vi "control v3.vi"(0 "Contraste":dbl, 1 "Ajuste ON?":bool=TRUE, 2 "Control ON?":bool=TRUE, 5 "Arreglo de Salida":dbl[](array[numeric]), 7 "Señal de Control IN":dbl[](array[numeric]), 9 "Parametros Actuales":T2, 11 "Parametros Iniciales":T2, 12 "Parametros Control":T3) -> (4 "Control Case OUT":T1 items=["00 - Promedio Inicial", "01 - Genera señal aleatoria", "02 - Incrementa t0", "03 - Promedia buen t0", "04 - Inicializa Amplitud", "05 - Incrementa Amplitud", "06 - Promedia buena Amplitud", "07 - Inicializa Sigma", "08 - Incrementa Sigma", "09 - Promedia buen Sigma", "10 - Actualiza mejor señal", "11 - Control ON, Ajuste OFF", "12 - Control OFF"], 6 "Contraste Promedio":dbl, 8 "Señal de Control OUT":dbl[](array[numeric]), 10 "Mejores Parametros OUT":T2)   [LabVIEW 2010]
uses:
  CaseControl.ctl
  <vilib>/Analysis/NI_AALBase.lvlib
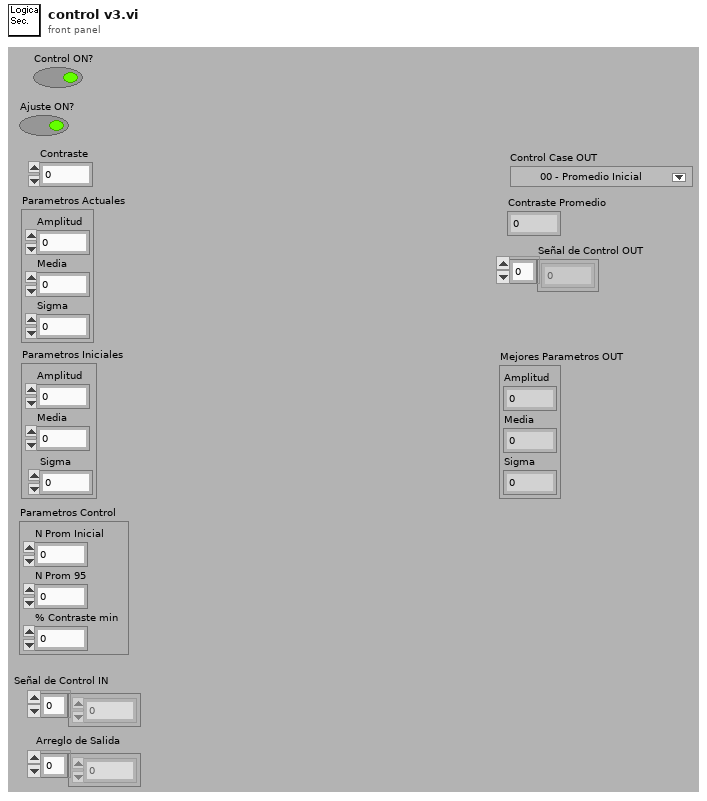
[diagram p1: front panel]
types:
  T1 = typedef "CaseControl.ctl" = u32
  T2 = cluster{"Amplitud":dbl, "Media":dbl, "Sigma":dbl}
  T3 = cluster{"N Prom Inicial":u32, "N Prom 95":u32, "% Contraste min":dbl}
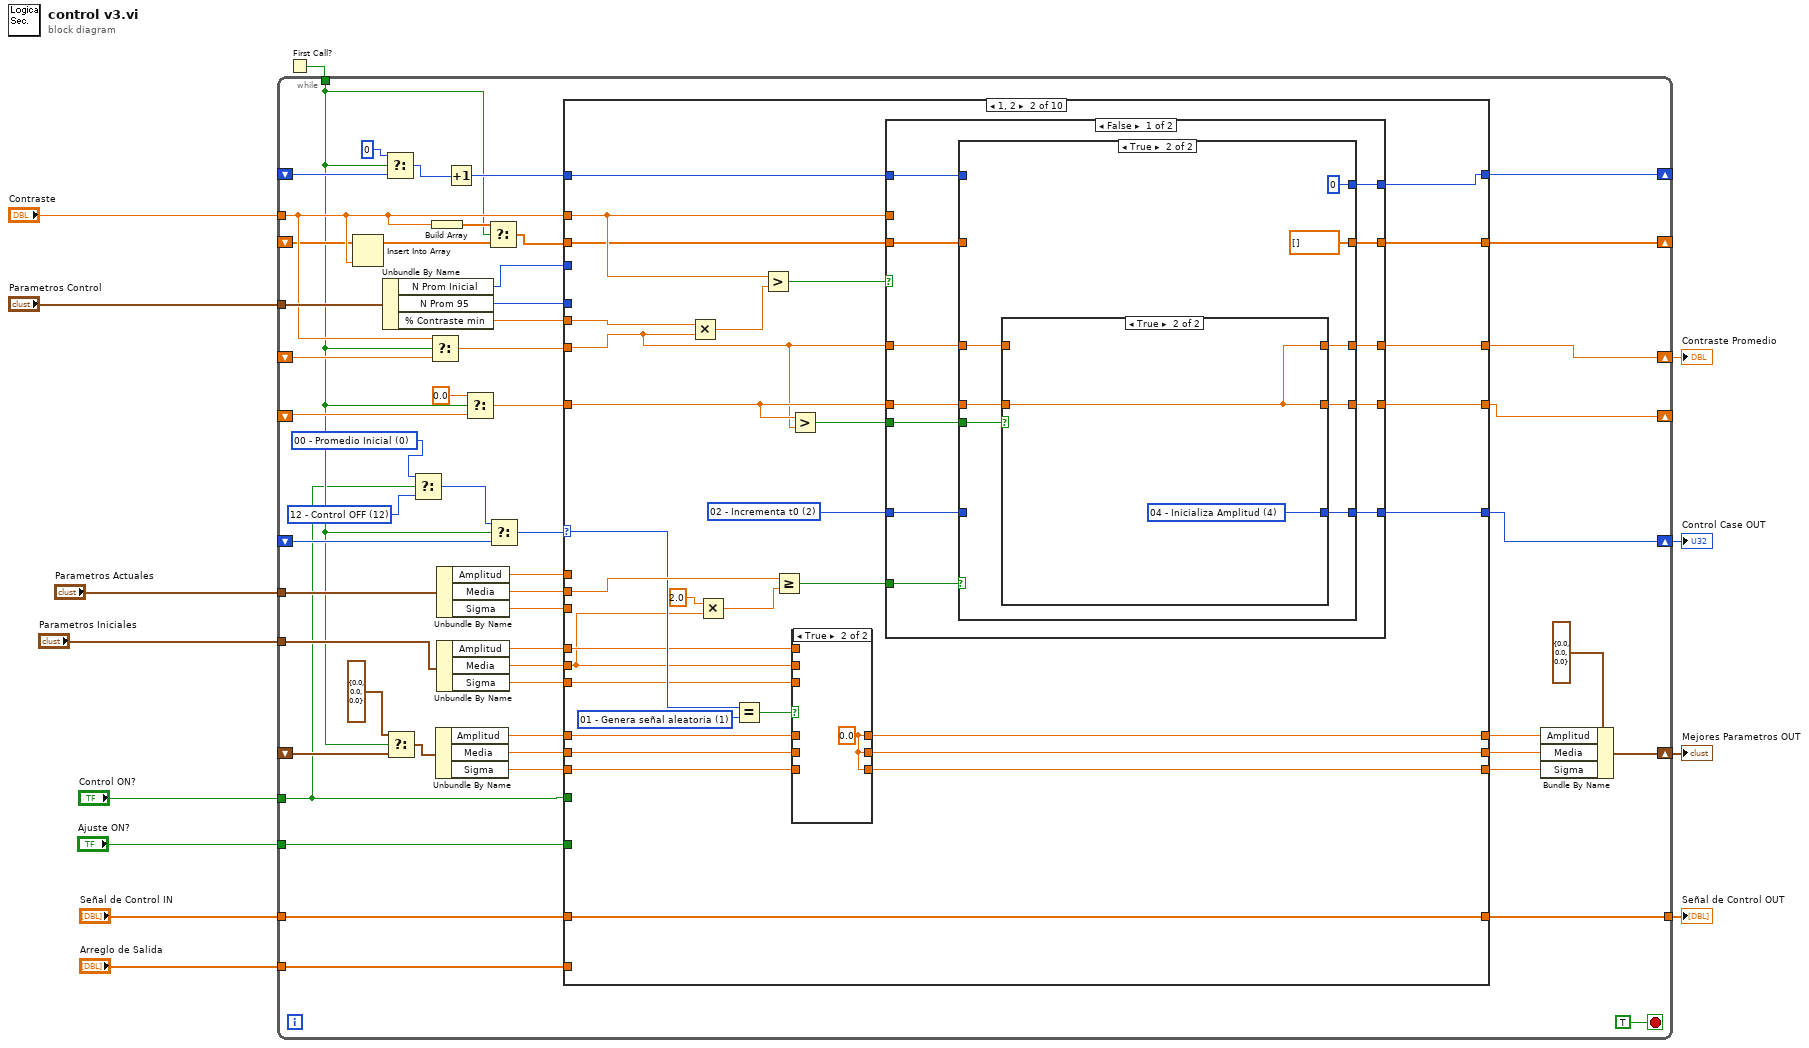
[diagram p0: block diagram]
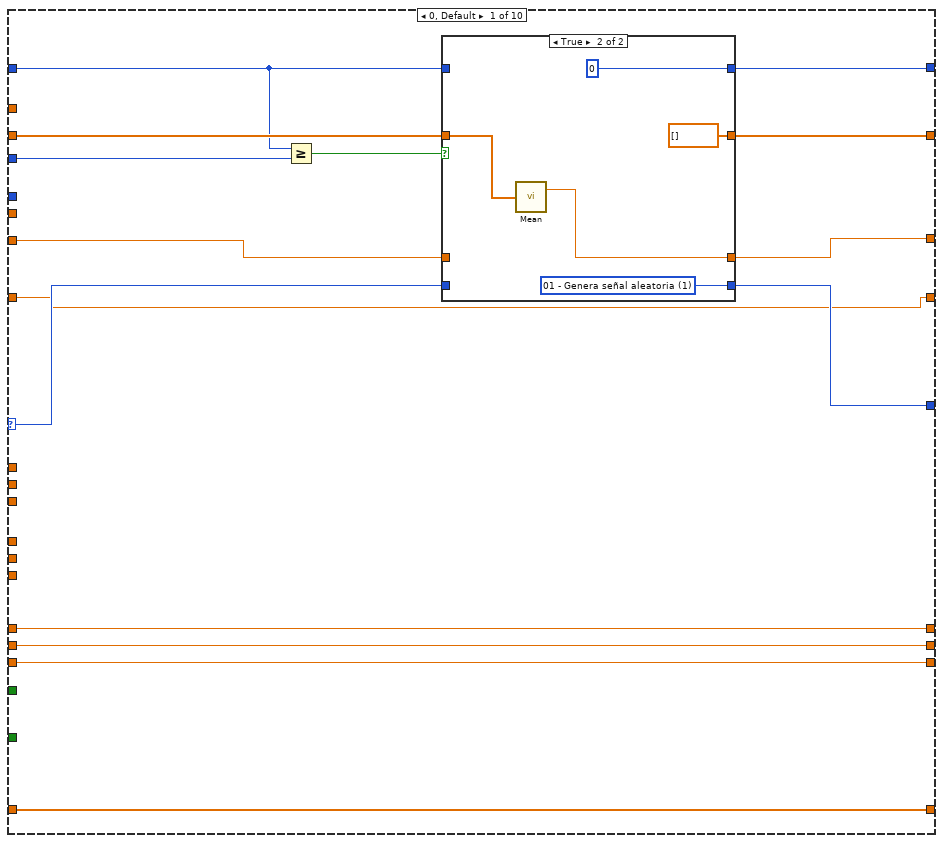
[diagram p2: hidden frame]
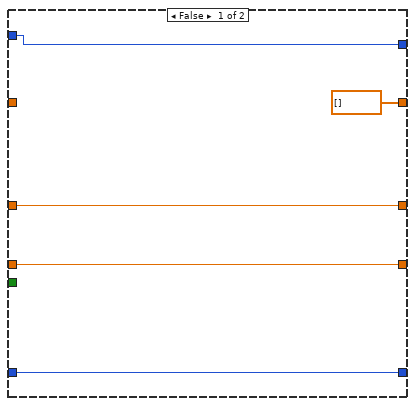
[diagram p5: hidden frame]
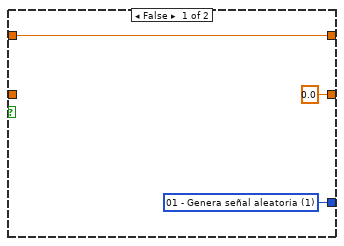
[diagram p6: hidden frame]
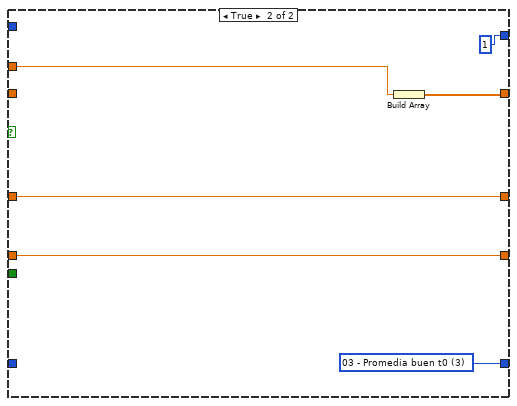
[diagram p7: hidden frame]
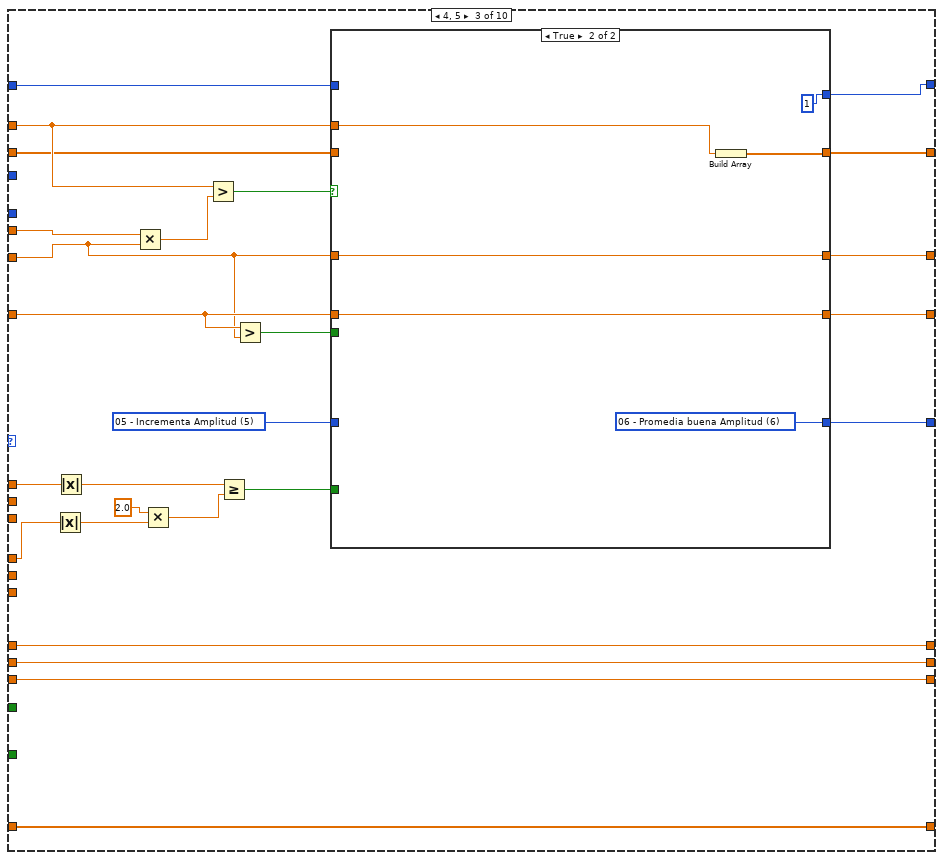
[diagram p8: hidden frame]
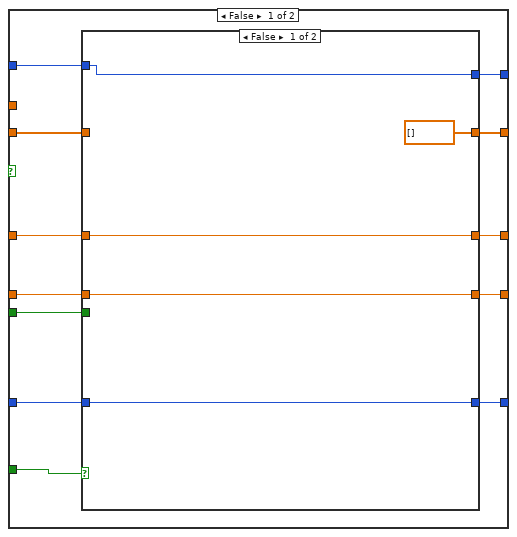
[diagram p9: hidden frame]
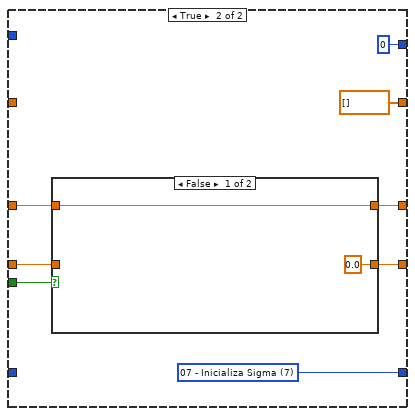
[diagram p10: hidden frame]
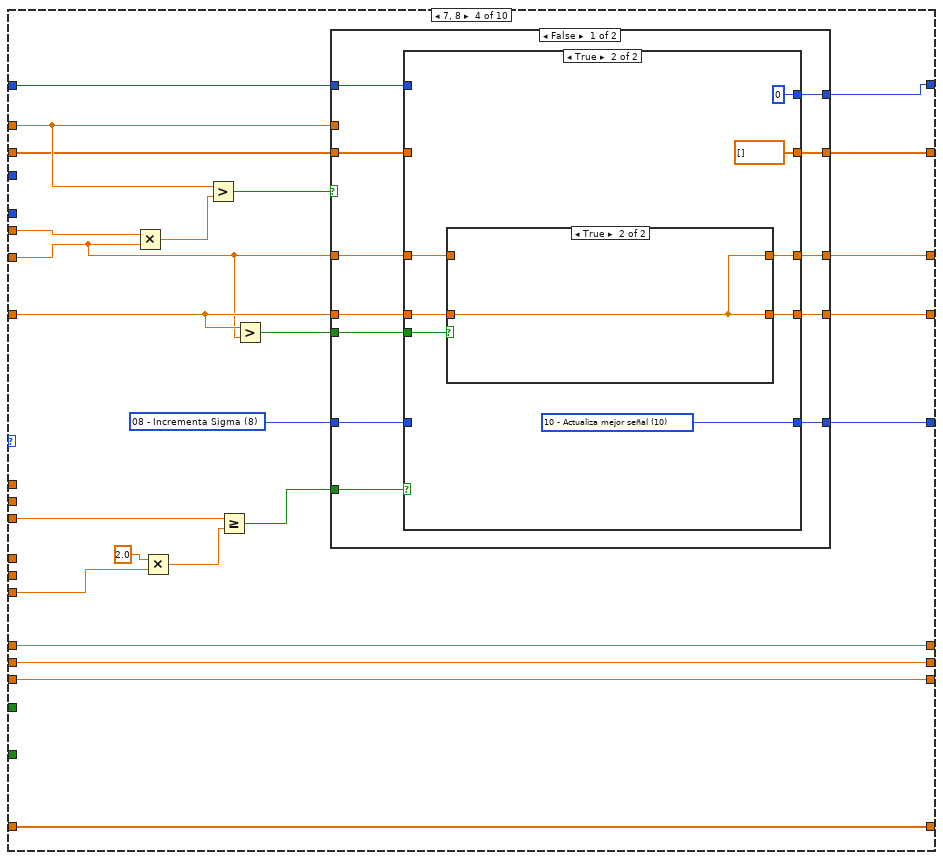
[diagram p12: hidden frame]
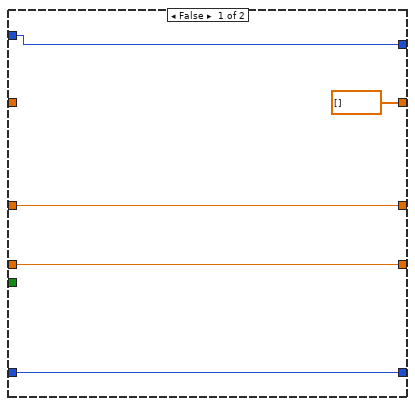
[diagram p13: hidden frame]
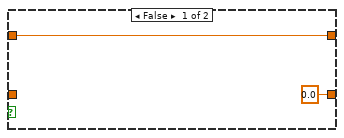
[diagram p14: hidden frame]
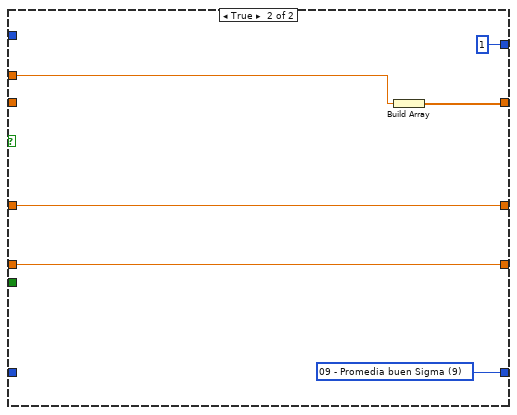
[diagram p15: hidden frame]
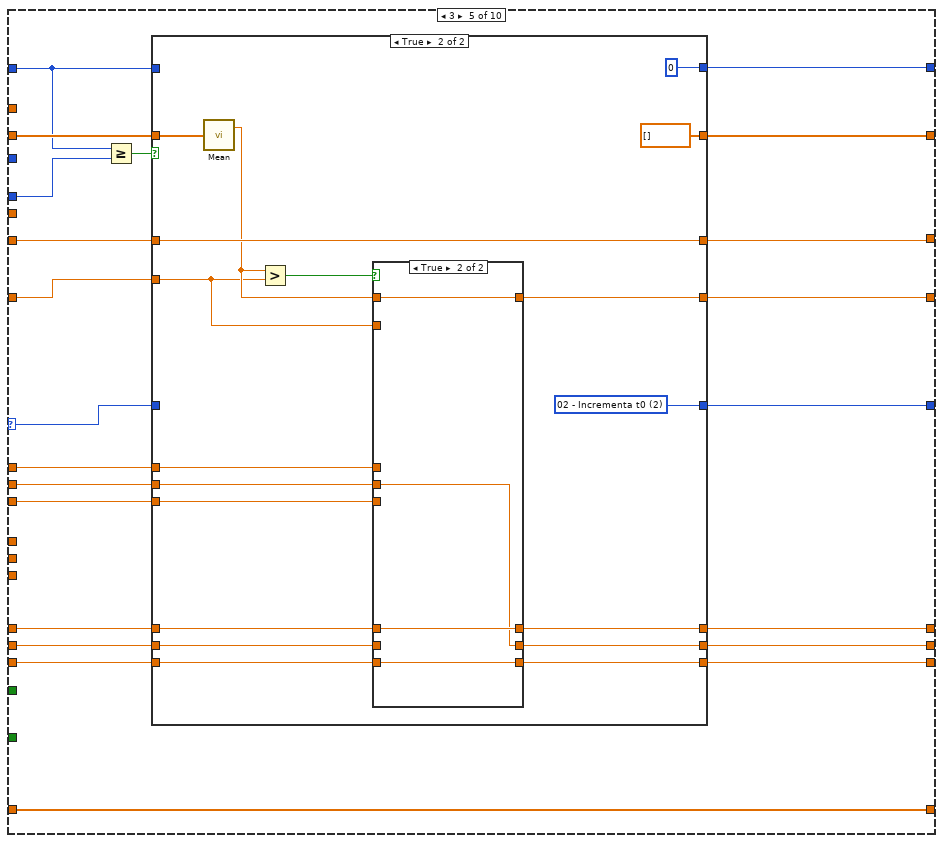
[diagram p16: hidden frame]
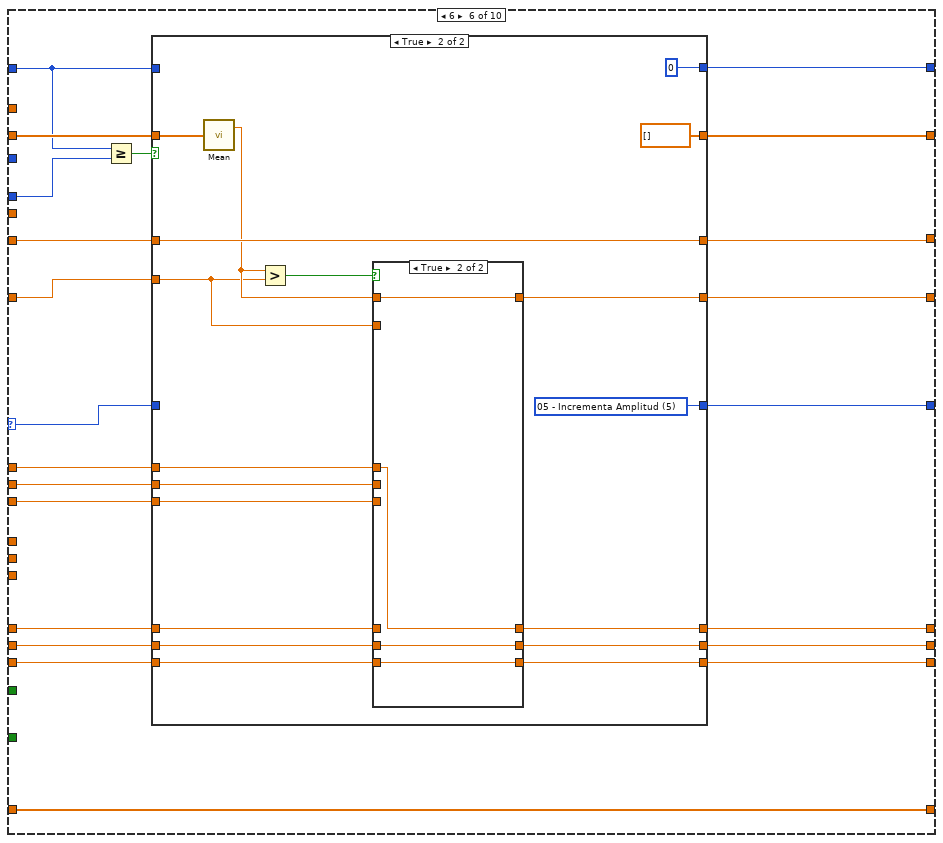
[diagram p19: hidden frame]
diagram:
  n1 = First Call?() -> (First Call?: T/F=w13:bool)
  n2 = while {
    tunnel: w13 -> [w22]
    tunnel: "Contraste" -> [w51]
    tunnel: "Parametros Control" -> [w66]
    shift-right: [w52] -> w3
    shift-left: _ -> [w54]
    shift-right: [w63] -> _
    shift-left: _ -> [w65]
    shift-right: [w60] -> _
    shift-left: _ -> [w48]
    shift-right: [w59] -> w2
    shift-left: _ -> [w58]
    tunnel: "Parametros Actuales" -> [w39]
    tunnel: "Parametros Iniciales" -> [w38]
    shift-right: [w34] -> w8
    shift-left: _ -> [w23]
    shift-right: [w26] -> _
    shift-left: _ -> [w29]
    tunnel: "Señal de Control IN" -> [w21]
    tunnel: "Arreglo de Salida" -> [w20]
    tunnel: [w19] -> w5
    tunnel: "Ajuste ON?" -> [w18]
    tunnel: "Control ON?" -> [w16]
    stop <- TRUE stop-if-true
    w14 = T1 0 items=["00 - Promedio Inicial", "01 - Genera señal aleatoria", "02 - Incrementa t0", "03 - Promedia buen t0", "04 - Inicializa Amplitud", "05 - Incrementa Amplitud", "06 - Promedia buena Amplitud", "07 - Inicializa Sigma", "08 - Incrementa Sigma", "09 - Promedia buen Sigma", "10 - Actualiza mejor señal", "11 - Control ON, Ajuste OFF", "12 - Control OFF"] ("f")
    w15 = T1 12 items=["00 - Promedio Inicial", "01 - Genera señal aleatoria", "02 - Incrementa t0", "03 - Promedia buen t0", "04 - Inicializa Amplitud", "05 - Incrementa Amplitud", "06 - Promedia buena Amplitud", "07 - Inicializa Sigma", "08 - Incrementa Sigma", "09 - Promedia buen Sigma", "10 - Actualiza mejor señal", "11 - Control ON, Ajuste OFF", "12 - Control OFF"] ("f")
    n3 = Insert Into Array(array=w48, new element=w51) -> (w49:dbl[])  [unwired: 1 in]
    n4 = Unbundle By Name(w66) -> ("N Prom Inicial"=w62:u32, "N Prom 95"=w47:u32, "% Contraste min"=w46:dbl)
    n5 = Select(t=u32 0, s=w22, f=w65) -> (s? t:f=w56:u32)
    n6 = Select(t=T2 {"Amplitud"=0.0, "Media"=0.0, "Sigma"=0.0} ("Parametros Iniciales 2"), s=w22, f=w23) -> (s? t:f=w25:T2)
    n7 = Select(t=w14, s=w16, f=w15) -> (s? t:f=w17:T1)
    n8 = Select(t=w51, s=w22, f=w58) -> (s? t:f=w57:dbl)
    n9 = Build Array(w51) -> (w61:dbl[])
    n10 = Unbundle By Name(w25) -> ("Amplitud"=w37:dbl, "Media"=w36:dbl, "Sigma"=w35:dbl)
    n11 = Unbundle By Name(w39) -> ("Amplitud"=w45:dbl, "Media"=w44:dbl, "Sigma"=w43:dbl)
    n12 = Unbundle By Name(w38) -> ("Amplitud"=w42:dbl, "Media"=w41:dbl, "Sigma"=w40:dbl)
    n13 = Increment(x=w56) -> (x+1=w55:u32)
    n14 = Select(t=0.0, s=w22, f=w29) -> (s? t:f=w27:dbl)
    n15 = Select(t=w61, s=w22, f=w49) -> (s? t:f=w50:dbl[])
    n16 = Select(t=w17, s=w22, f=w54) -> (s? t:f=w53:T1)
    n17 = case shown="1, 2" w53 {
      selector: w53 -> [w75 w103 _ _ w297 w353 w409 _ _ _]
      tunnel: w51 -> [_ w116 w182 w240 _ _ _ _ _ _]
      tunnel: [w77 w107 w174 w232 w300 w356 w412 u32 0 ("t") w467 u32 0 ("t")] -> w63
      tunnel: w62 -> [w82 _ _ _ _ _ _ _ _ _]
      tunnel: [w73 w117 w183 w241 w296 w352 w408 w455 w469 w481] -> w52
      tunnel: w50 -> [w81 w114 w180 w238 w302 w358 w414 w451 w466 w484]
      tunnel: [w74 w115 w181 w239 w301 w357 w413 w451 w466 w484] -> w60
      tunnel: [w78 w118 w184 w242 w293 w349 w405 w450 w465 w483] -> w59
      tunnel: w57 -> [w79 w110 w176 w234 w295 w351 w407 w450 _ _]
      tunnel: w55 -> [w76 w106 w173 w231 w299 w355 w411 _ w467 _]
      tunnel: w47 -> [_ _ _ _ w298 w354 w410 _ _ _]
      tunnel: w46 -> [_ w120 w186 w244 _ _ _ _ _ _]
      tunnel: w45 -> [_ _ w168 _ w292 w348 w404 _ _ _]
      tunnel: w44 -> [_ w108 _ _ w291 w347 w403 _ _ _]
      tunnel: w43 -> [_ _ _ w226 w290 w346 w402 _ _ _]
      tunnel: w42 -> [_ w98 w165 _ _ _ _ _ _ _]
      tunnel: w41 -> [_ w97 _ _ _ _ _ _ _ _]
      tunnel: w40 -> [_ w96 _ w225 _ _ _ _ _ _]
      tunnel: w37 -> [w71 w101 w171 w229 w289 w345 w401 w463 w474 w476]
      tunnel: w36 -> [w70 w100 w170 w228 w288 w344 w400 w462 w473 w477]
      tunnel: w35 -> [w69 w99 w169 w227 w287 w343 w399 w461 w472 w478]
      tunnel: [w71 w95 w171 w229 w285 w341 w397 w463 w474 w476] -> w32
      tunnel: [w70 w94 w170 w228 w283 w339 w395 w462 w473 w477] -> w31
      tunnel: [w69 w93 w169 w227 w284 w340 w396 w461 w472 w478] -> w30
      tunnel: w27 -> [w72 w111 w177 w235 w294 w350 w406 _ _ _]
      tunnel: [w72 w112 w178 w236 w286 w342 w398 0.0 ("mean") 0.0 ("t") 0.0 ("t")] -> w26
      tunnel: w21 -> [w68 w92 w164 w224 w282 w338 w394 w457 w475 w479]
      tunnel: w20 -> [_ _ _ _ _ _ _ w456 _ _]
      tunnel: [w68 w92 w164 w224 w282 w338 w394 w458 w475 w479] -> w19
      tunnel: w18 -> [_ _ _ _ _ _ _ w453 w468 _]
      tunnel: w16 -> [_ _ _ _ _ _ _ _ _ w480]
      frame 0, Default {
        n18 = Greater Or Equal?(x=w76, y=w82) -> (x >= y?=w80:bool)
        n19 = case shown="True" w80 {
          tunnel: w81 -> [w83 w88]
          tunnel: [w86 w91] -> w78
          tunnel: w79 -> [w86 _]
          tunnel: w76 -> [w85 _]
          tunnel: [w85 u32 0 ("t")] -> w77
          tunnel: [w84 w89] -> w73
          tunnel: w75 -> [w84 _]
          tunnel: [w83 dbl[] []] -> w74
          frame False {
          }
          frame True {
            w89 = T1 1 items=["00 - Promedio Inicial", "01 - Genera señal aleatoria", "02 - Incrementa t0", "03 - Promedia buen t0", "04 - Inicializa Amplitud", "05 - Incrementa Amplitud", "06 - Promedia buena Amplitud", "07 - Inicializa Sigma", "08 - Incrementa Sigma", "09 - Promedia buen Sigma", "10 - Actualiza mejor señal", "11 - Control ON, Ajuste OFF", "12 - Control OFF"] ("ControlCase")
            n20 = call <vilib>:"Mean.vi"("X"=w88) -> ("mean"=w91:dbl)  [unwired: 1 out]
          }
        }
      }
      frame 1, 2 {
        w102 = T1 1 items=["00 - Promedio Inicial", "01 - Genera señal aleatoria", "02 - Incrementa t0", "03 - Promedia buen t0", "04 - Inicializa Amplitud", "05 - Incrementa Amplitud", "06 - Promedia buena Amplitud", "07 - Inicializa Sigma", "08 - Incrementa Sigma", "09 - Promedia buen Sigma", "10 - Actualiza mejor señal", "11 - Control ON, Ajuste OFF", "12 - Control OFF"] ("y")
        w105 = T1 2 items=["00 - Promedio Inicial", "01 - Genera señal aleatoria", "02 - Incrementa t0", "03 - Promedia buen t0", "04 - Inicializa Amplitud", "05 - Incrementa Amplitud", "06 - Promedia buena Amplitud", "07 - Inicializa Sigma", "08 - Incrementa Sigma", "09 - Promedia buen Sigma", "10 - Actualiza mejor señal", "11 - Control ON, Ajuste OFF", "12 - Control OFF"] ("ControlCase")
        n21 = Multiply(x=w120, y=w110) -> (x*y=w119:dbl)
        n22 = Multiply(x=2.0, y=w97) -> (x*y=w122:dbl)
        n23 = Equal?(x=w103, y=w102) -> (x = y?=w104:bool)
        n24 = Greater?(x=w116, y=w119) -> (0:w121:bool)
        n25 = Greater Or Equal?(x=w108, y=w122) -> (x >= y?=w113:bool)
        n26 = Greater?(x=w111, y=w110) -> (0:w109:bool)
        n27 = case shown="True" w104 {
          tunnel: [w126 w127] -> w95
          tunnel: w101 -> [w126 _]
          tunnel: [w125 w127] -> w94
          tunnel: w100 -> [w125 _]
          tunnel: [w124 w127] -> w93
          tunnel: w99 -> [w124 _]
          tunnel: w98 -> [_ _]
          tunnel: w97 -> [_ _]
          tunnel: w96 -> [_ _]
          frame False {
          }
          frame True {
            w127 = 0.0 ("Amplitud")
          }
        }
        n28 = case shown="False" w121 {
          tunnel: [w134 w160] -> w118
          tunnel: w110 -> [w133 w160]
          tunnel: [w138 w163] -> w117
          tunnel: w105 -> [w137 _]
          tunnel: w116 -> [_ w161]
          tunnel: [w136 w162] -> w115
          tunnel: w114 -> [w135 _]
          tunnel: w113 -> [w139 _]
          tunnel: w111 -> [w132 w159]
          tunnel: [w131 w159] -> w112
          tunnel: w109 -> [w130 _]
          tunnel: [w129 u32 1] -> w107
          tunnel: w106 -> [w128 _]
          frame False {
            n29 = case shown="True" w139 {
              tunnel: [w144 w151] -> w138
              tunnel: w137 -> [w144 _]
              tunnel: [dbl[] [] dbl[] []] -> w136
              tunnel: w135 -> [_ _]
              tunnel: [w142 w150] -> w134
              tunnel: w133 -> [w142 w147]
              tunnel: w132 -> [w141 w149]
              tunnel: [w141 w148] -> w131
              tunnel: w130 -> [_ w152]
              tunnel: [w140 u32 0] -> w129
              tunnel: w128 -> [w140 _]
              frame False {
              }
              frame True {
                n30 = case shown="True" w152 {
                  tunnel: [w155 w157] -> w151
                  tunnel: [w154 w156] -> w150
                  tunnel: w149 -> [_ w156]
                  tunnel: [0.0 ("mean") w156] -> w148
                  tunnel: w147 -> [w154 _]
                  frame False {
                    w155 = T1 1 items=["00 - Promedio Inicial", "01 - Genera señal aleatoria", "02 - Incrementa t0", "03 - Promedia buen t0", "04 - Inicializa Amplitud", "05 - Incrementa Amplitud", "06 - Promedia buena Amplitud", "07 - Inicializa Sigma", "08 - Incrementa Sigma", "09 - Promedia buen Sigma", "10 - Actualiza mejor señal", "11 - Control ON, Ajuste OFF", "12 - Control OFF"] ("ControlCase")
                  }
                  frame True {
                    w157 = T1 4 items=["00 - Promedio Inicial", "01 - Genera señal aleatoria", "02 - Incrementa t0", "03 - Promedia buen t0", "04 - Inicializa Amplitud", "05 - Incrementa Amplitud", "06 - Promedia buena Amplitud", "07 - Inicializa Sigma", "08 - Incrementa Sigma", "09 - Promedia buen Sigma", "10 - Actualiza mejor señal", "11 - Control ON, Ajuste OFF", "12 - Control OFF"] ("ControlCase")
                  }
                }
              }
            }
          }
          frame True {
            w163 = T1 3 items=["00 - Promedio Inicial", "01 - Genera señal aleatoria", "02 - Incrementa t0", "03 - Promedia buen t0", "04 - Inicializa Amplitud", "05 - Incrementa Amplitud", "06 - Promedia buena Amplitud", "07 - Inicializa Sigma", "08 - Incrementa Sigma", "09 - Promedia buen Sigma", "10 - Actualiza mejor señal", "11 - Control ON, Ajuste OFF", "12 - Control OFF"] ("ControlCase")
            n31 = Build Array(w161) -> (w162:dbl[])
          }
        }
      }
      frame 4, 5 {
        w172 = T1 5 items=["00 - Promedio Inicial", "01 - Genera señal aleatoria", "02 - Incrementa t0", "03 - Promedia buen t0", "04 - Inicializa Amplitud", "05 - Incrementa Amplitud", "06 - Promedia buena Amplitud", "07 - Inicializa Sigma", "08 - Incrementa Sigma", "09 - Promedia buen Sigma", "10 - Actualiza mejor señal", "11 - Control ON, Ajuste OFF", "12 - Control OFF"] ("ControlCase")
        n32 = Absolute Value(x=w165) -> (abs(x)=w166:dbl)
        n33 = Absolute Value(x=w168) -> (abs(x)=w167:dbl)
        n34 = Multiply(x=w186, y=w176) -> (x*y=w185:dbl)
        n35 = Multiply(x=2.0, y=w166) -> (x*y=w188:dbl)
        n36 = Greater?(x=w182, y=w185) -> (0:w187:bool)
        n37 = Greater Or Equal?(x=w167, y=w188) -> (x >= y?=w179:bool)
        n38 = Greater?(x=w177, y=w176) -> (0:w175:bool)
        n39 = case shown="True" w187 {
          tunnel: [w196 w220] -> w184
          tunnel: w176 -> [w195 w220]
          tunnel: [w200 w223] -> w183
          tunnel: w172 -> [w199 _]
          tunnel: w182 -> [_ w221]
          tunnel: [w198 w222] -> w181
          tunnel: w180 -> [w197 _]
          tunnel: w179 -> [w201 _]
          tunnel: w177 -> [w194 w219]
          tunnel: [w193 w219] -> w178
          tunnel: w175 -> [w192 _]
          tunnel: [w191 u32 1] -> w174
          tunnel: w173 -> [w190 _]
          frame False {
            n40 = case shown="False" w201 {
              tunnel: [w206 w207] -> w200
              tunnel: w199 -> [w206 _]
              tunnel: [dbl[] [] dbl[] []] -> w198
              tunnel: w197 -> [_ _]
              tunnel: [w204 w213] -> w196
              tunnel: w195 -> [w204 w210]
              tunnel: w194 -> [w203 w212]
              tunnel: [w203 w211] -> w193
              tunnel: w192 -> [_ w214]
              tunnel: [w202 u32 0] -> w191
              tunnel: w190 -> [w202 _]
              frame False {
              }
              frame True {
                w207 = T1 7 items=["00 - Promedio Inicial", "01 - Genera señal aleatoria", "02 - Incrementa t0", "03 - Promedia buen t0", "04 - Inicializa Amplitud", "05 - Incrementa Amplitud", "06 - Promedia buena Amplitud", "07 - Inicializa Sigma", "08 - Incrementa Sigma", "09 - Promedia buen Sigma", "10 - Actualiza mejor señal", "11 - Control ON, Ajuste OFF", "12 - Control OFF"] ("ControlCase")
                n41 = case shown="False" w214 {
                  tunnel: [w216 w217] -> w213
                  tunnel: w212 -> [_ w217]
                  tunnel: [0.0 ("mean") w217] -> w211
                  tunnel: w210 -> [w216 _]
                  frame False {
                  }
                  frame True {
                  }
                }
              }
            }
          }
          frame True {
            w223 = T1 6 items=["00 - Promedio Inicial", "01 - Genera señal aleatoria", "02 - Incrementa t0", "03 - Promedia buen t0", "04 - Inicializa Amplitud", "05 - Incrementa Amplitud", "06 - Promedia buena Amplitud", "07 - Inicializa Sigma", "08 - Incrementa Sigma", "09 - Promedia buen Sigma", "10 - Actualiza mejor señal", "11 - Control ON, Ajuste OFF", "12 - Control OFF"] ("ControlCase")
            n42 = Build Array(w221) -> (w222:dbl[])
          }
        }
      }
      frame 7, 8 {
        w230 = T1 8 items=["00 - Promedio Inicial", "01 - Genera señal aleatoria", "02 - Incrementa t0", "03 - Promedia buen t0", "04 - Inicializa Amplitud", "05 - Incrementa Amplitud", "06 - Promedia buena Amplitud", "07 - Inicializa Sigma", "08 - Incrementa Sigma", "09 - Promedia buen Sigma", "10 - Actualiza mejor señal", "11 - Control ON, Ajuste OFF", "12 - Control OFF"] ("ControlCase")
        n43 = Multiply(x=w244, y=w234) -> (x*y=w243:dbl)
        n44 = Multiply(x=2.0, y=w225) -> (x*y=w246:dbl)
        n45 = Greater?(x=w240, y=w243) -> (0:w245:bool)
        n46 = Greater Or Equal?(x=w226, y=w246) -> (x >= y?=w237:bool)
        n47 = Greater?(x=w235, y=w234) -> (0:w233:bool)
        n48 = case shown="False" w245 {
          tunnel: [w254 w278] -> w242
          tunnel: w234 -> [w253 w278]
          tunnel: [w258 w281] -> w241
          tunnel: w230 -> [w257 _]
          tunnel: w240 -> [_ w279]
          tunnel: [w256 w280] -> w239
          tunnel: w238 -> [w255 _]
          tunnel: w237 -> [w259 _]
          tunnel: w235 -> [w252 w277]
          tunnel: [w251 w277] -> w236
          tunnel: w233 -> [w250 _]
          tunnel: [w249 u32 1] -> w232
          tunnel: w231 -> [w248 _]
          frame False {
            n49 = case shown="True" w259 {
              tunnel: [w264 w265] -> w258
              tunnel: w257 -> [w264 _]
              tunnel: [dbl[] [] dbl[] []] -> w256
              tunnel: w255 -> [_ _]
              tunnel: [w262 w271] -> w254
              tunnel: w253 -> [w262 w268]
              tunnel: w252 -> [w261 w270]
              tunnel: [w261 w269] -> w251
              tunnel: w250 -> [_ w272]
              tunnel: [w260 u32 0] -> w249
              tunnel: w248 -> [w260 _]
              frame False {
              }
              frame True {
                w265 = T1 10 items=["00 - Promedio Inicial", "01 - Genera señal aleatoria", "02 - Incrementa t0", "03 - Promedia buen t0", "04 - Inicializa Amplitud", "05 - Incrementa Amplitud", "06 - Promedia buena Amplitud", "07 - Inicializa Sigma", "08 - Incrementa Sigma", "09 - Promedia buen Sigma", "10 - Actualiza mejor señal", "11 - Control ON, Ajuste OFF", "12 - Control OFF"] ("ControlCase")
                n50 = case shown="True" w272 {
                  tunnel: [w274 w275] -> w271
                  tunnel: w270 -> [_ w275]
                  tunnel: [0.0 ("mean") w275] -> w269
                  tunnel: w268 -> [w274 _]
                  frame False {
                  }
                  frame True {
                  }
                }
              }
            }
          }
          frame True {
            w281 = T1 9 items=["00 - Promedio Inicial", "01 - Genera señal aleatoria", "02 - Incrementa t0", "03 - Promedia buen t0", "04 - Inicializa Amplitud", "05 - Incrementa Amplitud", "06 - Promedia buena Amplitud", "07 - Inicializa Sigma", "08 - Incrementa Sigma", "09 - Promedia buen Sigma", "10 - Actualiza mejor señal", "11 - Control ON, Ajuste OFF", "12 - Control OFF"] ("ControlCase")
            n51 = Build Array(w279) -> (w280:dbl[])
          }
        }
      }
      frame 3 {
        n52 = Greater Or Equal?(x=w299, y=w298) -> (x >= y?=w303:bool)
        n53 = case shown="True" w303 {
          tunnel: w302 -> [w310 w327]
          tunnel: w299 -> [w311 _]
          tunnel: [w311 u32 0 ("t")] -> w300
          tunnel: [w309 w328] -> w296
          tunnel: [w310 dbl[] []] -> w301
          tunnel: w297 -> [w309 _]
          tunnel: w295 -> [w308 w325]
          tunnel: w294 -> [w307 w312]
          tunnel: [w308 w325] -> w293
          tunnel: w292 -> [_ w323]
          tunnel: w291 -> [_ w322]
          tunnel: w290 -> [_ w321]
          tunnel: w289 -> [w306 w320]
          tunnel: w288 -> [w305 w319]
          tunnel: w287 -> [w304 w318]
          tunnel: [w307 w317] -> w286
          tunnel: [w306 w316] -> w285
          tunnel: [w304 w315] -> w284
          tunnel: [w305 w314] -> w283
          frame False {
          }
          frame True {
            w328 = T1 2 items=["00 - Promedio Inicial", "01 - Genera señal aleatoria", "02 - Incrementa t0", "03 - Promedia buen t0", "04 - Inicializa Amplitud", "05 - Incrementa Amplitud", "06 - Promedia buena Amplitud", "07 - Inicializa Sigma", "08 - Incrementa Sigma", "09 - Promedia buen Sigma", "10 - Actualiza mejor señal", "11 - Control ON, Ajuste OFF", "12 - Control OFF"] ("ControlCase")
            n54 = call <vilib>:"Mean.vi"("X"=w327) -> ("mean"=w313:dbl)  [unwired: 1 out]
            n55 = Greater?(x=w313, y=w312) -> (0:w324:bool)
            n56 = case shown="True" w324 {
              tunnel: w323 -> [_ _]
              tunnel: w322 -> [_ w335]
              tunnel: w321 -> [_ _]
              tunnel: w320 -> [w332 w337]
              tunnel: w319 -> [w331 _]
              tunnel: w318 -> [w330 w336]
              tunnel: [w333 w334] -> w317
              tunnel: [w332 w337] -> w316
              tunnel: [w330 w336] -> w315
              tunnel: [w331 w335] -> w314
              tunnel: w313 -> [_ w334]
              tunnel: w312 -> [w333 _]
              frame False {
              }
              frame True {
              }
            }
          }
        }
      }
      frame 6 {
        n57 = Greater Or Equal?(x=w355, y=w354) -> (x >= y?=w359:bool)
        n58 = case shown="True" w359 {
          tunnel: w358 -> [w366 w383]
          tunnel: w355 -> [w367 _]
          tunnel: [w367 u32 0 ("t")] -> w356
          tunnel: [w365 w384] -> w352
          tunnel: [w366 dbl[] []] -> w357
          tunnel: w353 -> [w365 _]
          tunnel: w351 -> [w364 w381]
          tunnel: w350 -> [w363 w368]
          tunnel: [w364 w381] -> w349
          tunnel: w348 -> [_ w379]
          tunnel: w347 -> [_ w378]
          tunnel: w346 -> [_ w377]
          tunnel: w345 -> [w362 w376]
          tunnel: w344 -> [w361 w375]
          tunnel: w343 -> [w360 w374]
          tunnel: [w363 w373] -> w342
          tunnel: [w362 w372] -> w341
          tunnel: [w360 w371] -> w340
          tunnel: [w361 w370] -> w339
          frame False {
          }
          frame True {
            w384 = T1 5 items=["00 - Promedio Inicial", "01 - Genera señal aleatoria", "02 - Incrementa t0", "03 - Promedia buen t0", "04 - Inicializa Amplitud", "05 - Incrementa Amplitud", "06 - Promedia buena Amplitud", "07 - Inicializa Sigma", "08 - Incrementa Sigma", "09 - Promedia buen Sigma", "10 - Actualiza mejor señal", "11 - Control ON, Ajuste OFF", "12 - Control OFF"] ("ControlCase")
            n59 = call <vilib>:"Mean.vi"("X"=w383) -> ("mean"=w369:dbl)  [unwired: 1 out]
            n60 = Greater?(x=w369, y=w368) -> (0:w380:bool)
            n61 = case shown="True" w380 {
              tunnel: w379 -> [_ w391]
              tunnel: w378 -> [_ _]
              tunnel: w377 -> [_ _]
              tunnel: w376 -> [w388 _]
              tunnel: w375 -> [w387 w390]
              tunnel: w374 -> [w386 w393]
              tunnel: [w389 w392] -> w373
              tunnel: [w388 w391] -> w372
              tunnel: [w386 w393] -> w371
              tunnel: [w387 w390] -> w370
              tunnel: w369 -> [_ w392]
              tunnel: w368 -> [w389 _]
              frame False {
              }
              frame True {
              }
            }
          }
        }
      }
      frame 9 {
        n62 = Greater Or Equal?(x=w411, y=w410) -> (x >= y?=w415:bool)
        n63 = case shown="True" w415 {
          tunnel: w414 -> [w422 w439]
          tunnel: w411 -> [w423 _]
          tunnel: [w423 u32 0 ("t")] -> w412
          tunnel: [w421 w440] -> w408
          tunnel: [w422 dbl[] []] -> w413
          tunnel: w409 -> [w421 _]
          tunnel: w407 -> [w420 w437]
          tunnel: w406 -> [w419 w424]
          tunnel: [w420 w437] -> w405
          tunnel: w404 -> [_ w435]
          tunnel: w403 -> [_ w434]
          tunnel: w402 -> [_ w433]
          tunnel: w401 -> [w418 w432]
          tunnel: w400 -> [w417 w431]
          tunnel: w399 -> [w416 w430]
          tunnel: [w419 w429] -> w398
          tunnel: [w418 w428] -> w397
          tunnel: [w416 w427] -> w396
          tunnel: [w417 w426] -> w395
          frame False {
          }
          frame True {
            w440 = T1 8 items=["00 - Promedio Inicial", "01 - Genera señal aleatoria", "02 - Incrementa t0", "03 - Promedia buen t0", "04 - Inicializa Amplitud", "05 - Incrementa Amplitud", "06 - Promedia buena Amplitud", "07 - Inicializa Sigma", "08 - Incrementa Sigma", "09 - Promedia buen Sigma", "10 - Actualiza mejor señal", "11 - Control ON, Ajuste OFF", "12 - Control OFF"] ("ControlCase")
            n64 = call <vilib>:"Mean.vi"("X"=w439) -> ("mean"=w425:dbl)  [unwired: 1 out]
            n65 = Greater?(x=w425, y=w424) -> (0:w436:bool)
            n66 = case shown="True" w436 {
              tunnel: w435 -> [_ _]
              tunnel: w434 -> [_ _]
              tunnel: w433 -> [_ w446]
              tunnel: w432 -> [w444 w447]
              tunnel: w431 -> [w443 w448]
              tunnel: w430 -> [w442 _]
              tunnel: [w445 w449] -> w429
              tunnel: [w444 w447] -> w428
              tunnel: [w442 w446] -> w427
              tunnel: [w443 w448] -> w426
              tunnel: w425 -> [_ w449]
              tunnel: w424 -> [w445 _]
              frame False {
              }
              frame True {
              }
            }
          }
        }
      }
      frame 10 {
        w452 = T1 11 items=["00 - Promedio Inicial", "01 - Genera señal aleatoria", "02 - Incrementa t0", "03 - Promedia buen t0", "04 - Inicializa Amplitud", "05 - Incrementa Amplitud", "06 - Promedia buena Amplitud", "07 - Inicializa Sigma", "08 - Incrementa Sigma", "09 - Promedia buen Sigma", "10 - Actualiza mejor señal", "11 - Control ON, Ajuste OFF", "12 - Control OFF"] ("f")
        w454 = T1 1 items=["00 - Promedio Inicial", "01 - Genera señal aleatoria", "02 - Incrementa t0", "03 - Promedia buen t0", "04 - Inicializa Amplitud", "05 - Incrementa Amplitud", "06 - Promedia buena Amplitud", "07 - Inicializa Sigma", "08 - Incrementa Sigma", "09 - Promedia buen Sigma", "10 - Actualiza mejor señal", "11 - Control ON, Ajuste OFF", "12 - Control OFF"] ("ControlCase")
        n67 = Add(x=w457, y=w456) -> (x+y=w458:dbl[])
        n68 = Select(t=w454, s=w453, f=w452) -> (s? t:f=w455:T1)
      }
      frame 11 {
        w470 = T1 11 items=["00 - Promedio Inicial", "01 - Genera señal aleatoria", "02 - Incrementa t0", "03 - Promedia buen t0", "04 - Inicializa Amplitud", "05 - Incrementa Amplitud", "06 - Promedia buena Amplitud", "07 - Inicializa Sigma", "08 - Incrementa Sigma", "09 - Promedia buen Sigma", "10 - Actualiza mejor señal", "11 - Control ON, Ajuste OFF", "12 - Control OFF"] ("f")
        w471 = T1 1 items=["00 - Promedio Inicial", "01 - Genera señal aleatoria", "02 - Incrementa t0", "03 - Promedia buen t0", "04 - Inicializa Amplitud", "05 - Incrementa Amplitud", "06 - Promedia buena Amplitud", "07 - Inicializa Sigma", "08 - Incrementa Sigma", "09 - Promedia buen Sigma", "10 - Actualiza mejor señal", "11 - Control ON, Ajuste OFF", "12 - Control OFF"] ("ControlCase")
        n69 = call <vilib>:"Mean.vi"("X"=w466) -> ("mean"=w465:dbl)  [unwired: 1 out]
        n70 = Select(t=w471, s=w468, f=w470) -> (s? t:f=w469:T1)
      }
      frame 12 {
        w486 = T1 12 items=["00 - Promedio Inicial", "01 - Genera señal aleatoria", "02 - Incrementa t0", "03 - Promedia buen t0", "04 - Inicializa Amplitud", "05 - Incrementa Amplitud", "06 - Promedia buena Amplitud", "07 - Inicializa Sigma", "08 - Incrementa Sigma", "09 - Promedia buen Sigma", "10 - Actualiza mejor señal", "11 - Control ON, Ajuste OFF", "12 - Control OFF"] ("f")
        w487 = T1 0 items=["00 - Promedio Inicial", "01 - Genera señal aleatoria", "02 - Incrementa t0", "03 - Promedia buen t0", "04 - Inicializa Amplitud", "05 - Incrementa Amplitud", "06 - Promedia buena Amplitud", "07 - Inicializa Sigma", "08 - Incrementa Sigma", "09 - Promedia buen Sigma", "10 - Actualiza mejor señal", "11 - Control ON, Ajuste OFF", "12 - Control OFF"] ("ControlCase")
        n71 = call <vilib>:"Mean.vi"("X"=w484) -> ("mean"=w483:dbl)  [unwired: 1 out]
        n72 = Select(t=w487, s=w480, f=w486) -> (s? t:f=w481:T1)
      }
    }
    n73 = Bundle By Name(cluster=T2 {"Amplitud"=0.0, "Media"=0.0, "Sigma"=0.0} ("Parametros Iniciales 2"), "Amplitud"=w32, "Media"=w31, "Sigma"=w30) -> (w34:T2)
  }
  "Mejores Parametros OUT" <- w8
  "Señal de Control OUT" <- w5
  "Control Case OUT" <- w3
  "Contraste Promedio" <- w2
